vi "dfd_Build Indent.vi"(11 "indent order":i32) -> (3 "tag indent":string)   [LabVIEW 2017, in "NI_DigFilter_Process.lvlib"]
uses:
  <vilib>/addons/Digital Filter Design/NI_DigFilter_Process.lvlib
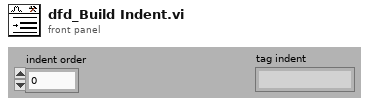
[diagram p1: front panel]
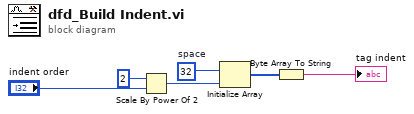
[diagram p0: block diagram]
diagram:
  w2 = u8 32  # space
  n1 = Scale By Power Of 2(n=2, x="indent order") -> (x*2^n=w3:i32)
  n2 = Initialize Array(w2, w3) -> (w1:u8[])
  n3 = Byte Array To String(unsigned byte array=w1) -> (string=→"tag indent":string)
